vi "About LabActor.vi"(8 "Error In":errorcluster) -> (0 "Error Out":errorcluster)   [LabVIEW 2025]
panel:
  out "Last modified":string
  out "Build version":string
  # "LabActor Framework"
  # "© 2012-2025\n\nFedor F. Balakirev\nfbalakirev@gmail.com"
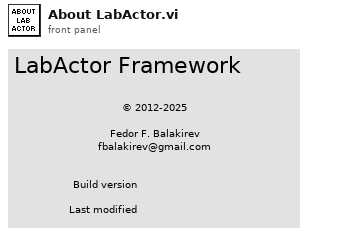
[diagram p1: front panel]
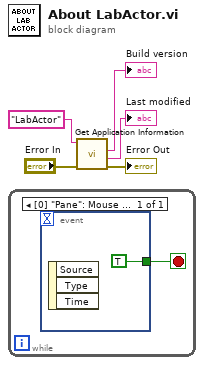
[diagram p0: block diagram]
diagram:
  n1 = while {
    stop <- w6 stop-if-true
    n2 = event shown="[0] \"Pane\": Mouse Down;  Key Down;  Panel Close" {
      selector: _ -> [_]
      dyn-events: _ -> [_]
      timeout: _ -> [_]
      tunnel: [TRUE] -> w6
      event Mouse Down; Key Down; Panel Close {
        n3 = event-data() -> ()  [unwired: 1 in, 3 out]
      }
    }
  }
  n4 = call "Get Application Information.vi"("error out"="Error In", "Build Name"="LabActor") -> ("Error Out"=→"Error Out":errorcluster, "Last modified"=→"Last modified":string, "Build version"=→"Build version":string)  [unwired: 5 in, 2 out]
